vi "Dashboard Main.vi"() -> ()   [LabVIEW 2015]
uses:
  Common Code/Auton Command Cluster.ctl
  Common Code/Auton File Lists.ctl
  Vision/Camera Types.ctl
  Common Code/Goal Vision Packet.ctl
  <vilib>/Rock Robotics/WPI/Camera/WPI_CameraSettings Read MJPG.ctl
  <vilib>/Rock Robotics/WPI/Camera/WPI_CameraImageSize.ctl
  Common Code/Encoder Values Super Cluster.ctl
  Common Code/Encoder Values.ctl
  Common Code/Power and Diagnostic Data.ctl
  Common Code/Utilities/PDP Data.ctl
  Common Code/Utilities/PCM Data.ctl
  Common Code/IMU Data.ctl
  navX-MXP Library/COMMON/TypeDefs/Value TypeDefs/navX NAVX_CAL_STATUS.ctl
  navX-MXP Library/COMMON/TypeDefs/Value TypeDefs/navX NAVX_OP_STATUS.ctl
  Common Code/Intake Status Cluster.ctl
  Common Code/Intake Mode.ctl
  Common Code/Intake States.ctl
  Common Code/Climb Status Cluster.ctl
  Common Code/Climb Mode.ctl
  Common Code/Climb Presets.ctl
  Common Code/Major Loop Times.ctl
  Common Code/Shooter State Cluster.ctl
  Common Code/Shooter State.ctl
  Common Code/Shoot Modes Enum.ctl
  Common Code/Shot Type.ctl
  Common Code/Encoder Control.ctl
  Common Code/Drivetrain Status Cluster.ctl
  Common Code/Drivetrain Modes.ctl
  Common Code/Dist Drive Status.ctl
  Common Code/Drivetrain Settings.ctl
  Common Code/Shooter Presets.ctl
  Common Code/Shot Presets.ctl
  Common Code/Intake Presets.ctl
  Common Code/Drivetrain Output Range.ctl
  Common Code/Enabled Systems.ctl
  Common Code/Ultrasonic Data.ctl
  Common Code/Autonomous Presets.ctl
  Common Code/Robot Name.ctl
  Common Code/Dashboard Communication/Dashboard Control Data.ctl
  Common Code/Dashboard Drivetrain Command.ctl
  Common Code/Drivetrain Vision.ctl
  Common Code/Ball Tracking Command Cluster.ctl
  Common Code/Ball Vision Packet.ctl
  Common Code/Tracking Mode.ctl
  Common Code/IntakeEcoderControl.ctl
  Common Code/Dashboard Communication/Dashboard Display Data.ctl
  <vilib>/Rock Robotics/WPI/Dashboard/WPI_DashboardLogging Global.vi
  <vilib>/Utility/inputDevices.llb/keyboardAcquire.vi
  navX-MXP Library/navX-MXP IMU.lvlib
panel:
  in  "Robot":T1
  in  "Logging Filename":path=path ""
  in  "stop":bool
  out "DumbDashMessage":string="137 values loaded OK"
  in  "Save":bool
  in  "Load":bool
  in  "TCP":refnum<k5>
  in  "Rec Mode":enum32{"Stop", "Record", "Playback"}(radio)
  out "Image Message":string="Timeout in Camera Communications"
  in  "Dashboard Tab":T2(tab)
  out "Front Camera Display 2":T3(plugin-control)
  out "Pressure":dbl
  out "Goal Active? 2":bool
  out "Drivetrain Mode":bool
  out "Intake State":bool
  out "Right RPM":dbl(knob) scale=0.0..5000.0
  out "Left RPM":dbl(knob) scale=0.0..5000.0
  out "Mode":T4(ring)=enum."Disconnected"
  out "Shooter Mode":bool
  out "Gyro":dbl(knob) scale=0.0..360.0 scale format="%#.7g"
  out "Climb Mode":bool
  out "Intake Mode":bool
  out "Shooter State":bool
  out "Camera IP":string="0.0.0.0"
  out "Robot IP":string="0.0.0.0"
  out "Angle Ready?":bool
  out "RPM Ready?":bool
  out "Vision Ready?":bool
  out "Ball Loaded?":bool
  out "Shooter Ready?":bool
  out "Front Camera Display":T3(plugin-control)
  in  "Camera Mode":u16(ring)=3 items=["Camera Off", "USB Camera SW", "USB Camera HW", "IP Camera"]
  out "FPS":dbl
  out "Bandwidth (Mbps)":dbl
  out "NAVX_CAL_STATUS":T5 items=["IMU_CAL_STATE_MASK"=3, "IMU_CAL_INPROGRESS"=0, "IMU_CAL_ACCUMULATE"=1, "IMU_CAL_COMPLETE"=2, "MAG_CAL_COMPLETE"=4, "BARO_CAL_COMPLETE"=8]
  in  "Auton Presets":T6
  out "Auton Command Cluster":T7
  out "Auton File Lists":T8
  in  "Drivetrain Settings":T9={"Gyro Tolerance"=6.0, "Throttle Ramp (ms)"=250.0, "Angular rate compensation"=FALSE, "Throttle to Rate Scale"=0.0, "Rate compensation gain"=0.0, "Kv"=0.0, "Ka"=0.0, "Feed Forward P"=1.0, "Feed Forward D"=0.0, "Goal Vision PID gains"={"proportional gain (Kc)"=0.8, "integral time (Ti, min)"=0.05, "derivative time (Td, min)"=0.003}, "Goal Detection Window"=12.0, "Creep Rate"=0.0} {"Goal Vision PID gains"."derivative time (Td, min)" format="%.3f"; "Goal Vision PID gains"."integral time (Ti, min)" format="%.3f"; "Goal Vision PID gains"."proportional gain (Kc)" format="%.4f"}
  out "Drivetrain Status Cluster":T10 {"2nd Gear Time" scale=0.0..135.0; "1st Gear Time" scale=0.0..135.0}
  in  "Encoder Settings":T13={"Right Tick Constant"=0.002781, "Left Tick Constant"=0.002785, "Reset?"=FALSE, "Y Dist"={"PID gains"={"proportional gain (Kc)"=0.0, "integral time (Ti, min)"=0.0, "derivative time (Td, min)"=0.0}}, "Y Stop Thresh"=0.0, "Y Stop Speed"=0.0}
  in  "Goal Output Range":cluster{"output high":dbl, "output low":dbl}={"output high"=0.8, "output low"=-0.8}
  out "Encoder Values":T14
  in  "Steer PID output":cluster{"output high":dbl, "output low":dbl}
  in  "Steer PID gains":T16
  in  "Shooter Presets":T17={"Batter Shot"={"Left"=1450.0, "Right"=1450.0, "Angle"=69.0}, "Deep Middle Shot"={"Left"=0.0, "Right"=0.0, "Angle"=0.0}, "Manual Shot"={"Left"=1000.0, "Right"=1000.0, "Angle"=0.0}, "Left Ticks Per Rotation"=-409.6, "Right Ticks Per Rotation"=409.6, "Low Bar Shot"={"Left"=2100.0, "Right"=2100.0, "Angle"=42.0}, "Shooter RPM Tolerance"=100.0, "IIR Filter Power"=0.0, "Trigger Power"=0.9, "Fire from Load Delay"=250, "Max Angle"=80.0, "Min Angle"=42.0, "Angle PID gains"={"P"=1.0, "I"=0.0, "D"=0.002}, "Angle Output"={"output high"=0.5, "output low"=-0.5}, "Shooter Angle Tolerance"=3.0, "Vision Shoot x^2"=0.0, "Vision Shoot x"=0.0, "Offset Angle"=0.0, "High Goal Center Height"=97.0, "Feed Forward Max Accel"=160.57, "Feed Forward Kv"=0.000217, "Backwards Trigger"=-0.6, "Shot Finish Delay (ms)"=250.0, "Angle Max Current"=40.0, "Angle Current Trip Time"=500.0, "Intake Angle"=80.0, "Vision Shoot c"=0.0, "Reset?"=FALSE, "Servo Release Delay"=0.0, "Servo Idle Angle"=120, "Servo Hold Angle"=55, "Angle Pot x"=7.0746, "Angle Pot c"=33.439, "Ignore Angle?"=FALSE, "Manual Output?"=FALSE, "Manual Out"=0.0, "Max RPM"=4600.0, "Safty Frist Angle"=44.0, "Intake Danger Height"=35.0, "Angle Pot B"=0, "Angle Pot M"=12.0, "FF Finish RPM"=0.0, "RPM PID Right"={"P"=0.17, "I"=0.0, "D"=0.0, "FF"=0.036}, "RPM PID Left"={"P"=0.18, "I"=0.0, "D"=0.0, "FF"=0.037}, "Backwards RPM"=-300.0, "Vision RPM"=0.0} {"Angle Output"."output low" format="%.2f"; "Angle Output"."output high" format="%.2f"}
  out "Shooter State Cluster":T19 {"Trigger Output" scale=-1.0..1.0; "Angle Motor Output" scale=-1.0..1.0; "Right RPM" scale=0.0..5000.0; "Left RPM" scale=0.0..5000.0}
  in  "Intake Presets":T23={"Intake Speed"=0.8, "Outake Speed"=-0.8, "Low Height"=5.0, "Half Height"=55.0, "Full Height"=90.0, "Angle Speed"=0.0, "Angle Tolerance"=5.0, "Encoder Scale"=0.001478, "Load Height"=4.0, "Output Range"={"output high"=0.4, "output low"=-0.4}, "Rotation Power Max/Min"=0.5, "MaxCurrent"=40.0, "Intake Trip Time"=500.0, "Idle Height"=27.0, "Max Height"=90.0, "Reset Encoders?"=FALSE, "PID gains"={"proportional gain (Kc)"=1.0, "integral time (Ti, min)"=0.0, "derivative time (Td, min)"=0.003}} {"Max Height" format="%#_7g"; "Idle Height" format="%#_7g"; "Intake Trip Time" format="%#_7g"; "MaxCurrent" format="%#_7g"; "Rotation Power Max/Min" format="%#_7g"; "Load Height" format="%#_7g"; "Encoder Scale" format="%#_7g"; "Angle Tolerance" format="%#_7g"; "Angle Speed" format="%#_7g"; "Full Height" format="%#_7g"; "Half Height" format="%#_7g"; "Low Height" format="%#_7g"; "Outake Speed" format="%#_7g"; "Intake Speed" format="%#_7g"}
  out "Intake Status Cluster":T25
  in  "Climb Presets":T28={"Pull Power"=0.0, "Time to Hold"=0.0, "Extend Power"=1.0}
  out "Climb Status Cluster":T29
  in  "Pressure B":dbl
  in  "Pressure M":dbl=22.0
  out "Pressure Sensor Voltage":dbl
  out "IMU Data":T31 {"NAVX_OP_STATUS" items=["INITIALIZING", "SELFTEST_IN_PROGRESS", "ERROR", "IMU_AUTOCAL_IN_PROGRESS", "NORMAL"]; "NAVX_CAL_STATUS" items=["IMU_CAL_STATE_MASK"=3, "IMU_CAL_INPROGRESS"=0, "IMU_CAL_ACCUMULATE"=1, "IMU_CAL_COMPLETE"=2, "MAG_CAL_COMPLETE"=4, "BARO_CAL_COMPLETE"=8]}
  out "Gyro 2":dbl(knob) scale=0.0..360.0 scale format="%#.7g"
  out "Ultrasonic Data":T33
  out "Ball Cam Active?":bool
  out "Camera Display 2":T3(plugin-control)
  in  "Aspect Fudge Factor":dbl=1.0
  in  "Score Threshold 2":dbl=75.0 format="%#_13g"
  out "Goal Display":T3(plugin-control)
  out "Found Targets":T34(array[cluster]) {"Normalized Rect"."Numeric 5" format="%#_2g"; "Normalized Rect"."Numeric 3" format="%#_2g"; "Normalized Rect"."Numeric 2" format="%#_2g"; "Normalized Rect"."Numeric" format="%#_2g"}
  in  "Camera Type":T35=enum."1013"
  out "Goal Vision Packet":T36
  in  "Goal Camera Settings":T37={"fps"=30, "compression"=30, "Image Size"=enum."320x240"}
  in  "File number":i32
  in  "Use Goal File?":bool
  in  "Color Components":T39={"Hue"={110.0, 142.0}, "Sat"={138.0, 255.0}, "Val"={139.0, 198.0}} {"Val" scale=0.0..255.0; "Sat" scale=0.0..255.0; "Hue" scale=0.0..255.0 scale format="%#_3g"}
  out "Goal Active?":bool
  in  "Camera Mode 2":u16(ring) items=["Camera Off", "USB Camera SW", "USB Camera HW", "IP Camera"]
  out "FPS 2":dbl
  out "Bandwidth (Mbps) 2":dbl
  in  "Ball Camera Settings":T37={"fps"=30, "compression"=30, "Image Size"=enum."320x240"}
  out "Front Camera Display 3":T3(plugin-control)
  out "Power and Diagnostic Data":T40
  in  "Enabled Systems":T43={"Shoot"=TRUE, "Intake"=TRUE, "DT"=TRUE, "Gyro"=TRUE, "100ms"=TRUE, "US"=TRUE}
  out "Control Info":T44
  out "Status Info":T45
  out "DS TCP":T46={"Error Strings"="", "Disable Counts"={0, 0}, "Rail Faults"={0, 0, 0}, "Robot IP"="0.0.0.0", "DB Mode"=4, "Event Info"={"Name"="", "Type"=0, "Number"=0, "Replay"=0}, "Camera Addr"="0.0.0.0"}
  out "Robot Metrics":T47
  out "Loop Times":T48
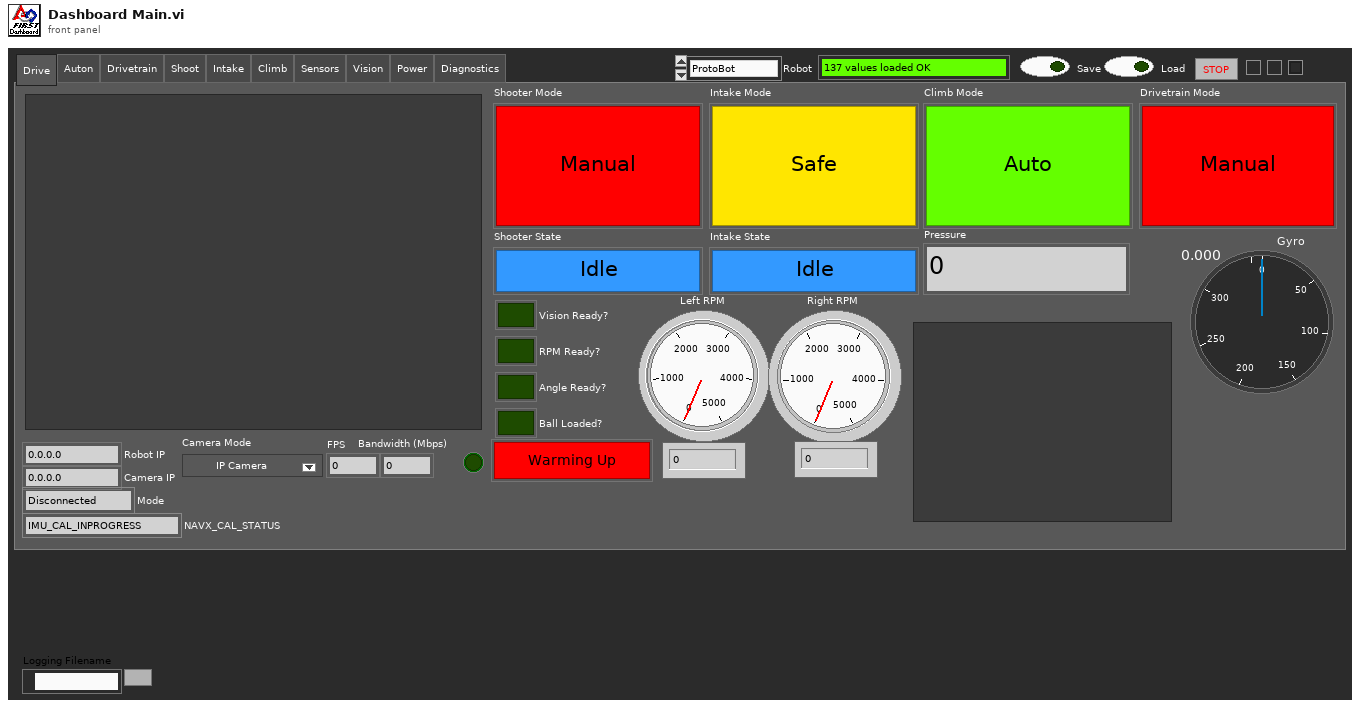
[diagram p1: front panel]
types:
  T1 = typedef "Robot Name.ctl" = enum16{"ProtoBot", "Main Robot", "Practice Robot"}
  T2 = enum32{"Drive", "Auton", "Drivetrain", "Shoot", "Intake", "Climb", "Sensors", "Vision", "Power", "Diagnostics"}
  T3 = typedef "IMAQ Image.ctl" = refnum<image>
  T4 = enum8{"Tele-Op Disabled", "Tele-Op Enabled", "Auto Disabled", "Auto Enabled", "Test Disabled", "Test Enabled", "Disconnected", "No Code", "E-Stop"}
  T5 = typedef "navX-MXP IMU.lvlib/navX NAVX_CAL_STATUS.ctl" = u8
  T6 = typedef "Autonomous Presets.ctl" = cluster{"Pitch Limit":dbl, "Roll Limit":dbl, "Ultrasonic Limit":dbl, "Start Position":dbl, "Cross Position":dbl}
  T7 = typedef "Auton Command Cluster.ctl" = cluster{"Command ID":i32, "maxTime":dbl, "Y Distance":dbl, "Heading":dbl, "Throttle":dbl, "Async":dbl, "Velocity":dbl, "Acceleration":dbl, "To":dbl, "Condition":dbl, "Shot Type":dbl, "Left RPM":dbl, "Override RPM":i32, "Override Angle":i32, "Right RPM":dbl, "Angle":dbl, "Intake Mode":i32, "Intake Cmd":i32, "Intake O":i32, "Eject O":i32, "Angle O":i32, "Arm O":i32, "Intake Speed":dbl, "Eject Speed":dbl, "Arm Angle":dbl, "Arm Speed":dbl, "Intake?":i32, "Eject?":i32, "Left":dbl, "Right":dbl, "Pivot Speed":dbl}
  T8 = typedef "Auton File Lists.ctl" = cluster{"Current Queue":string, "General Scripts":string, "Defense Scripts":string, "Movement Scripts":string}
  T9 = typedef "Drivetrain Settings.ctl" = cluster{"Gyro Tolerance":dbl, "Throttle Ramp (ms)":dbl, "Angular rate compensation":bool, "Throttle to Rate Scale":dbl, "Rate compensation gain":dbl, "Kv":dbl, "Ka":dbl, "Feed Forward P":dbl, "Feed Forward D":dbl, "Goal Vision PID gains":cluster{"proportional gain (Kc)":dbl, "integral time (Ti, min)":dbl, "derivative time (Td, min)":dbl}, "Goal Detection Window":dbl, "Creep Rate":dbl}
  T10 = typedef "Drivetrain Status Cluster.ctl" = cluster{"Modes":T11, "Y (Throttle)":dbl, "X (Steer)":dbl, "Gyro In Range?":bool, "Distance Drive Finished?":bool, "Stop Eject Lockout":bool, "Dist Drive Status":T12, "Y Target":dbl, "Heading Target":dbl, "Vision Target Aligned?":bool, "Gear":dbl, "1st Gear Time":dbl, "2nd Gear Time":dbl, "1st Gear Shifts":dbl, "2nd Gear Shifts":dbl}
  T11 = typedef "Drivetrain Modes.ctl" = enum16{"Tank", "Climb", "Manual", "Goal Vision Targeting", "PID Distance Drive", "Hybrid", "Gyro Steer"}
  T12 = typedef "Dist Drive Status.ctl" = cluster{"Y In Range":bool, "X In Range":bool, "Gyro In Range":bool, "Y Dist":dbl, "X Dist":dbl, "Gyro":dbl}
  T13 = typedef "Encoder Control.ctl" = cluster{"Right Tick Constant":dbl, "Left Tick Constant":dbl, "Reset?":bool, "Y Dist":cluster{"PID gains":cluster{"proportional gain (Kc)":dbl, "integral time (Ti, min)":dbl, "derivative time (Td, min)":dbl}}, "Y Stop Thresh":dbl, "Y Stop Speed":dbl}
  T14 = typedef "Encoder Values Super Cluster.ctl" = cluster{"Left Encoder":T15, "Right Encoder":T15}
  T15 = typedef "Encoder Values.ctl" = cluster{"Distance":dbl, "Speed":dbl, "Ticks":dbl}
  T16 = cluster{"proportional gain (Kc)":dbl, "integral time (Ti, min)":dbl, "derivative time (Td, min)":dbl}
  T17 = typedef "Shooter Presets.ctl" = cluster{"Batter Shot":T18, "Deep Middle Shot":T18, "Manual Shot":T18, "Left Ticks Per Rotation":dbl, "Right Ticks Per Rotation":dbl, "Low Bar Shot":T18, "Shooter RPM Tolerance":dbl, "IIR Filter Power":dbl, "Trigger Power":dbl, "Fire from Load Delay":i32, "Max Angle":dbl, "Min Angle":dbl, "Angle PID gains":cluster{"P":dbl, "I":dbl, "D":dbl}, "Angle Output":cluster{"output high":dbl, "output low":dbl}, "Shooter Angle Tolerance":dbl, "Vision Shoot x^2":dbl, "Vision Shoot x":dbl, "Offset Angle":dbl, "High Goal Center Height":dbl, "Feed Forward Max Accel":dbl, "Feed Forward Kv":dbl, "Backwards Trigger":dbl, "Shot Finish Delay (ms)":dbl, "Angle Max Current":dbl, "Angle Current Trip Time":dbl, "Intake Angle":dbl, "Vision Shoot c":dbl, "Reset?":bool, "Servo Release Delay":dbl, "Servo Idle Angle":i32, "Servo Hold Angle":i32, "Angle Pot x":dbl, "Angle Pot c":dbl, "Ignore Angle?":bool, "Manual Output?":bool, "Manual Out":dbl, "Max RPM":dbl, "Safty Frist Angle":dbl, "Intake Danger Height":dbl, "Angle Pot B":i32, "Angle Pot M":dbl, "FF Finish RPM":dbl, "RPM PID Right":cluster{"P":dbl, "I":dbl, "D":dbl, "FF":dbl}, "RPM PID Left":cluster{"P":dbl, "I":dbl, "D":dbl, "FF":dbl}, "Backwards RPM":dbl, "Vision RPM":dbl}
  T18 = typedef "Shot Presets.ctl" = cluster{"Left":dbl, "Right":dbl, "Angle":dbl}
  T19 = typedef "Shooter State Cluster.ctl" = cluster{"State":T20, "Left RPM":dbl, "Right RPM":dbl, "Shooter Ready?":bool, "Ball Loaded?":bool, "Current Angle":dbl, "Angle Motor Output":dbl, "Trigger Output":dbl, "Angle Ready?":bool, "RPM Ready?":bool, "Vision Ready?":bool, "Ball Loaded?":bool, "Mode":T21, "Shot Type":T22, "Pot Height":dbl, "Current Tripped Forward?":bool, "Current Tripped Backward?":bool, "Right Servo":i32, "Left Servo":i32, "IR Override":bool, "Intake Danger?":bool}
  T20 = typedef "Shooter State.ctl" = enum16{"Idle", "Warmup", "Shooter Ready", "Shoot"}
  T21 = typedef "Shoot Modes Enum.ctl" = enum16{"Manual", "Safe", "Auto"}
  T22 = typedef "Shot Type.ctl" = enum16{"Batter Shot", "Corner Shot", "Curve Shot", "Vision Shot", "Deep Middle Shot"}
  T23 = typedef "Intake Presets.ctl" = cluster{"Intake Speed":dbl, "Outake Speed":dbl, "Low Height":dbl, "Half Height":dbl, "Full Height":dbl, "Angle Speed":dbl, "Angle Tolerance":dbl, "Encoder Scale":dbl, "Load Height":dbl, "Output Range":T24, "Rotation Power Max/Min":dbl, "MaxCurrent":dbl, "Intake Trip Time":dbl, "Idle Height":dbl, "Max Height":dbl, "Reset Encoders?":bool, "PID gains":cluster{"proportional gain (Kc)":dbl, "integral time (Ti, min)":dbl, "derivative time (Td, min)":dbl}}
  T24 = typedef "Drivetrain Output Range.ctl" = cluster{"output high":dbl, "output low":dbl}
  T25 = typedef "Intake Status Cluster.ctl" = cluster{"Roller Power":dbl, "Angle Power":dbl, "Intake Mode":T26, "Intake States":T27, "Rollers Active?":bool, "Current Height":dbl, "Target Height":dbl, "Encoder Raw Position":dbl, "Forward Tripped?":bool, "Backward Tripped?":bool, "Override IR?":bool}
  T26 = typedef "Intake Mode.ctl" = enum16{"Safe", "Auto", "Manual"}
  T27 = typedef "Intake States.ctl" = enum16{"Idle", "Set roller speed", "Move to angle"}
  T28 = typedef "Climb Presets.ctl" = cluster{"Pull Power":dbl, "Time to Hold":dbl, "Extend Power":dbl}
  T29 = typedef "Climb Status Cluster.ctl" = cluster{"Pull Power":dbl, "Unpin Power":dbl, "PTO Engaged?":bool, "Climb Mode":T30}
  T30 = typedef "Climb Mode.ctl" = enum16{"Auto", "Semi-Auto", "Manual"}
  T31 = typedef "IMU Data.ctl" = cluster{"Pitch":sgl, "Roll":sgl, "Yaw":sgl, "Data Valid?":bool, "Temp":sgl, "MOVING":bool, "YAW_STABLE":bool, "Accel X":sgl, "Accel Y":sgl, "Accel Z":sgl, "Accel Magnitude":sgl, "Pitch Rate":sgl, "Roll Rate":sgl, "Yaw Rate":sgl, "NavX Opened?":bool, "NAVX_CAL_STATUS":T5, "NAVX_OP_STATUS":T32}
  T32 = typedef "navX-MXP IMU.lvlib/navX NAVX_OP_STATUS.ctl" = u8
  T33 = typedef "Ultrasonic Data.ctl" = cluster{"Left Ultrasonic":dbl, "Right Ultrasonic":dbl}
  T34 = cluster{"Distance (ft)":dbl, "Center":cluster{dbl, dbl}, "Normalized Rect":cluster{"Numeric":dbl, "Numeric 2":dbl, "Numeric 3":dbl, "Numeric 5":dbl}}[]
  T35 = typedef "Camera Types.ctl" = enum16{"206", "1011", "1013", "MS HD3000 square", "MS HD3000 640x480"}
  T36 = typedef "Goal Vision Packet.ctl" = cluster{"Distance":dbl, "Center X":dbl, "Center Y":dbl, "Found Target?":bool, "Robot Center":dbl, "Angle":dbl}
  T37 = typedef "WPI_CameraSettings Read MJPG.ctl" = cluster{"fps":i32, "compression":i32, "Image Size":T38}
  T38 = typedef "WPI_CameraImageSize.ctl" = enum16{"640x480", "320x240", "160x120", "Custom"}
  T39 = cluster{"Hue":cluster{dbl, dbl}, "Sat":cluster{dbl, dbl}, "Val":cluster{dbl, dbl}}
  T40 = typedef "Power and Diagnostic Data.ctl" = cluster{"PDP Data":T41, "PCM Data":T42, "roboRIO input voltage (V)":dbl, "roboRIO input current (A)":dbl, "3.3V Rail Short":bool, "5 V Rail Short":bool, "6 V Rail Short":bool, "roboRIO Brownout":bool, "Outputs Enabled?":bool}
  T41 = typedef "PDP Data.ctl" = cluster{"Battery Voltage":sgl, "Temperature (degrees C)":sgl, "Internal Battery R (Ohms)":sgl, "Energy (J)":sgl, "Power (W)":sgl, "Total Current (A)":sgl, "Battery Voltage Fault":bool, "Temperature Fault":bool, "Hardware Fault":bool, "Currents":cluster{"[0]":sgl, "[1]":sgl, "[2]":sgl, "[3]":sgl, "[4]":sgl, "[5]":sgl, "[6]":sgl, "[7]":sgl, "[8]":sgl, "[9]":sgl, "[10]":sgl, "[11]":sgl, "[12]":sgl, "[13]":sgl, "[14]":sgl, "[15]":sgl}, "Current Faults":cluster{"[0]":bool, "[1]":bool, "[2]":bool, "[3]":bool, "[4]":bool, "[5]":bool, "[6]":bool, "[7]":bool, "[8]":bool, "[9]":bool, "[10]":bool, "[11]":bool, "[12]":bool, "[13]":bool, "[14]":bool, "[15]":bool}}
  T42 = typedef "PCM Data.ctl" = cluster{"Compressor Fault":bool, "Solenoid Fault":bool, "Compressor Enabled":bool, "Hardware Fault":bool, "Compressor Current":dbl}
  T43 = typedef "Enabled Systems.ctl" = cluster{"Shoot":bool, "Intake":bool, "DT":bool, "Gyro":bool, "100ms":bool, "US":bool}
  T44 = cluster{"Control Bits":cluster{"TestMode":bool, "Autonomous":bool, "Enabled":bool, "FMS Present":bool, bool, bool, bool, "E-Stop":bool}, "Team Station ":u8, "Countdown":sgl, "Joystick Values":cluster{"Axes":dbl[], "Buttons":bool[], "POVs":i16[]}[]}
  T45 = cluster{"Status bits":cluster{"Test Mode":bool, "Autonomous":bool, "Enabled":bool, "Code Start":bool, "Brownout":bool, "Reserved 2":bool, "Reserved 3":bool, "E-Stop":bool}, "Code Trace":cluster{"Disabled":bool, "TeleOp":bool, "Auto":bool, "Test":bool}, "Controller Type":enum16{"unknown", "cRIO", "roboRio"}, "Code?":enum16{"unknown", "noCode", "code"}, "Battery V":dbl}
  T46 = cluster{"Error Strings":string, "Disable Counts":cluster{u16, u16}, "Rail Faults":cluster{u16, u16, u16}, "Robot IP":string, "DB Mode":u8, "Event Info":cluster{"Name":string, "Type":u8, "Number":u16, "Replay":u8}, "Camera Addr":string}
  T47 = cluster{"Storage":cluster{"Disk Free":u64, "RAM Block":u32, "RAM free":u32}, "CPU Utilization":cluster{"CPU % ISR":sgl, "CPU % Time Crit":sgl, "CPU % Timed Str":sgl, "CPU % High":sgl, "CPU % Above":sgl, "CPU % Normal":sgl, "CPU % Low":sgl}, "CAN":cluster{"% Bus Utilization":sgl, "Bus Off Cnt":u32, "TX_FIFO Full Cnt":u32, "Receive Error Cnt":u8, "Transmit Error Cnt":u8}, "HID":cluster{"HID Outputs":u32, "Rumble Low":u16, "Rumble High":u16}[]}
  T48 = typedef "Major Loop Times.ctl" = cluster{"DT Loop Timer":u32, "Shooter Loop Timer":u32, "Intake Loop Timer":u32, "US Loop Timer":u32, "Auton File Loop Timer":u32}
  T49 = typedef "Image Type" = u32
  T50 = typedef "NI_LVConfig.lvlib/Config Data RefNum.ctl" = refnum<k1>
  T51 = cluster{cluster{dbl, dbl}, cluster{dbl, dbl}, cluster{dbl, dbl}}
  T52 = cluster{"Bounding box":cluster{"left":dbl, "top":dbl, "right":dbl, "bottom":dbl}, "Aspect Ratio":dbl, "Area to CH":dbl, "X Mask":dbl, "Y Mask":dbl, "Moment":dbl}[]
  T53 = cluster{"Distance (ft)":dbl, "Center":cluster{dbl, dbl}, "Normalized Rect":cluster{"Numeric":dbl, "Numeric 2":dbl, "Numeric 3":dbl, "Numeric 5":dbl}}
  T54 = typedef "Dashboard Display Data.ctl" = cluster{"Auton Command Cluster":T7, "Auton File Lists":T8, "Drivetrain Status Cluster":T10, "Encoder Values":T14, "IMU Data":T31, "Power and Diagnostic Data":T40, "Gyro":dbl, "Shooter State Cluster":T19, "Intake Status Cluster":T25, "Ultrasonic Data":T33, "Climb Status Cluster":T29, "Loop Times":T48, "Pressure":dbl, "Pressure Voltage":dbl}
  T55 = typedef "Dashboard Control Data.ctl" = cluster{"Shooter Presets":T17, "Encoder Control":T13, "Steer PID output":cluster{"output high":dbl, "output low":dbl}, " Steer PID gains":cluster{"proportional gain (Kc)":dbl, "integral time (Ti, min)":dbl, "derivative time (Td, min)":dbl}, "Drivetrain Settings":T9, "Vision Packet":T36, "Dashboard Drivetrain Command":T56, "Info/Command Cluster":T58, "Ball Vision Packet":T59, "Intake Presets":T23, "Intake Encoder Control":T61, "Climb Presets":T28, "Goal Output Range":cluster{"output high":dbl, "output low":dbl}, "Enabled Systems":T43, "Auton Presets":T6, "Pressure M":dbl, "Pressure B":dbl}
  T56 = typedef "Dashboard Drivetrain Command.ctl" = cluster{"Drivetrain Vision":T57}
  T57 = typedef "Drivetrain Vision.ctl" = cluster{"Goal Window":dbl, "Ball Window":dbl}
  T58 = typedef "Ball Tracking Command Cluster.ctl" = cluster{"Distance to Ball":dbl, "Desired Angle":dbl, "Command":enum16{"Turn to Ball", "Turn to Angle", "Get Distance"}, "Pixels from Center":dbl}
  T59 = typedef "Ball Vision Packet.ctl" = cluster{"Ball Detected?":bool, "Distance to Ball":dbl, "Desired Angle":dbl, "Pixels from Center":dbl, "Tracking mode":T60}
  T60 = typedef "Tracking Mode.ctl" = enum16{"Turn to Ball", "Turn to Angle"}
  T61 = typedef "IntakeEcoderControl.ctl" = cluster{"Arm Tick Constant":dbl, "Reset?":bool, "Y Dist":cluster{"PID gains":cluster{"proportional gain (Kc)":dbl, "integral time (Ti, min)":dbl, "derivative time (Td, min)":dbl}}, "Y Stop Thresh":dbl, "Y Stop Speed":dbl}
  T62 = cluster{"Image Size":bool, "Image Type":bool, "Pixel Value":bool, "ROI Information":bool, "Zoom Factor":bool}
  T63 = enum16{"0", "1", "2", "3", "4", "5", "6", "7", "8", "9", "A", "B", "C", "D", "E", "F", "G", "H", "I", "J", "K", "L", "M", "N", "O", "P", "Q", "R", "S", "T", "U", "V", "W", "X", "Y", "Z", "F1", "F2", "F3", "F4", "F5", "F6", "F7", "F8", "F9", "F10", "F11", "F12", "F13", "F14", "F15", "ADD", "BACK", "BACKSLASH", "CAPITAL", "COMMA", "DECIMAL", "DELETE", "DIVIDE", "DOWN", "END", "EQUALS", "ESCAPE", "GRAVE (`)", "HOME", "INSERT", "LBRACKET", "LCONTROL", "LEFT", "L ALT", "LSHIFT", "LWIN", "MINUS", "MULTIPLY", "NEXT", "NUMLOCK", "NUMPAD_0", "NUMPAD_1", "NUMPAD_2", "NUMPAD_3", "NUMPAD_4", "NUMPAD_5", "NUMPAD_6", "NUMPAD_7", "NUMPAD_8", "NUMPAD_9", "PAUSE", "PERIOD", "PRIOR (PG UP)", "RBRACKET", "RCONTROL", "RETURN", "RIGHT", "R ALT", "RSHIFT", "RWIN", "SCROLL", "SEMICOLON", "SLASH", "SPACE", "SUBTRACT", "TAB", "UP", "ENTER (num pad)", "' (quote)"}[]
  T64 = typedef "DumbDash Control.ctl" = cluster{"Name":string, "Ref":refnum<vi>, "Type":T65}
  T65 = typedef "DumbDash Control Type.ctl" = enum16{"Invalid", "Number", "Boolean", "String"}
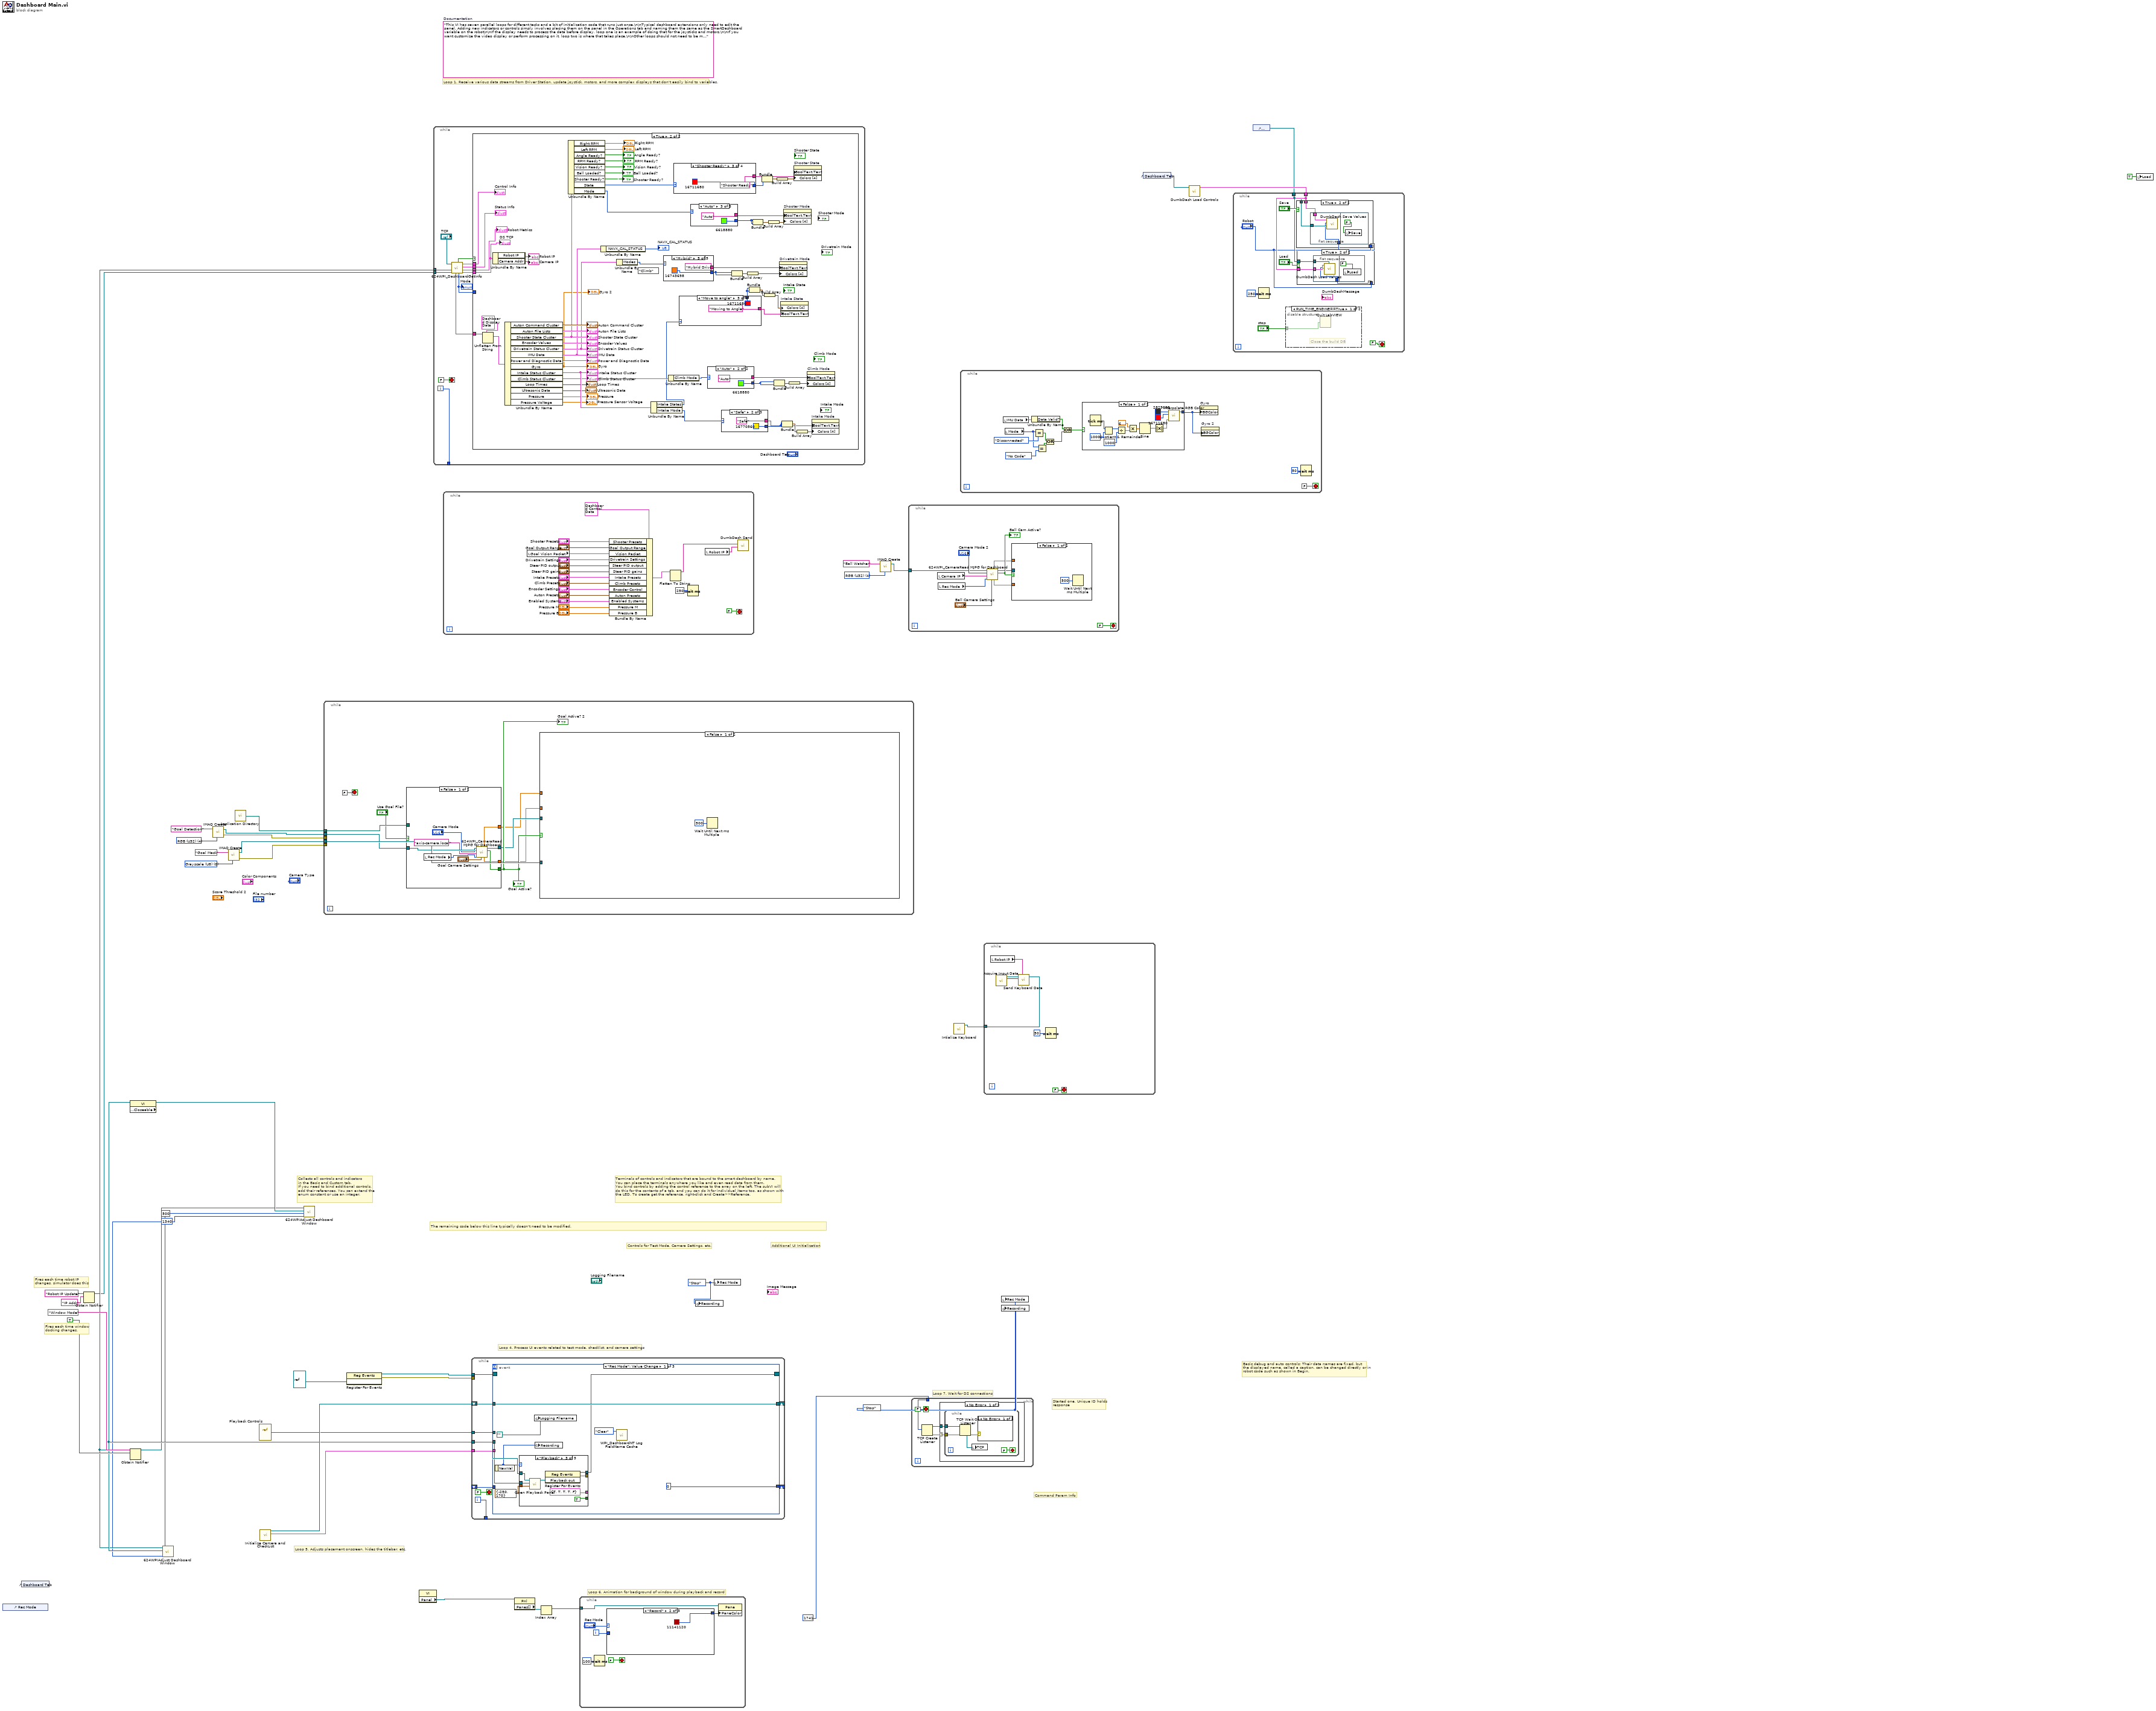
[diagram p0: block diagram]
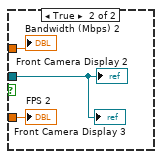
[diagram p2: hidden frame]
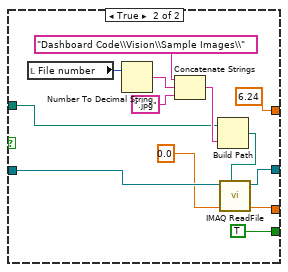
[diagram p3: hidden frame]
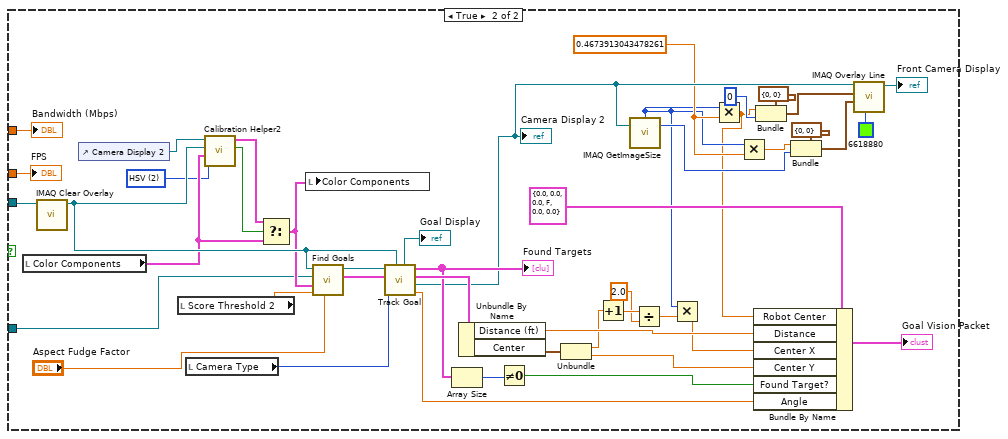
[diagram p4: hidden frame]
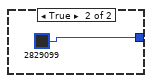
[diagram p5: hidden frame]
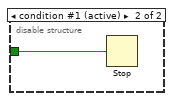
[diagram p6: hidden frame]
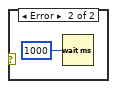
[diagram p9: hidden frame]
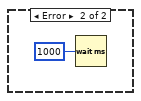
[diagram p10: hidden frame]
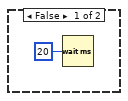
[diagram p11: hidden frame]
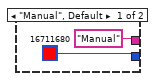
[diagram p12: hidden frame]
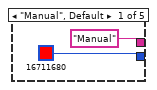
[diagram p13: hidden frame]
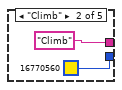
[diagram p14: hidden frame]
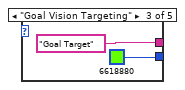
[diagram p15: hidden frame]
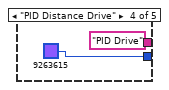
[diagram p16: hidden frame]
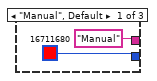
[diagram p17: hidden frame]
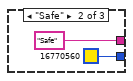
[diagram p18: hidden frame]
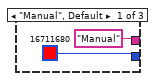
[diagram p19: hidden frame]
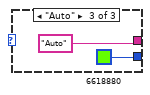
[diagram p20: hidden frame]
diagram:
  w4 = T49 4 items=["Grayscale (U8)", "Grayscale (I16)", "Grayscale (SGL)", "Complex (CSG)", "RGB (U32)", "HSL (U32)", "RGB (U64)", "Grayscale (U16)"] ("Image Type")
  w6 = T49 0 items=["Grayscale (U8)", "Grayscale (I16)", "Grayscale (SGL)", "Complex (CSG)", "RGB (U32)", "HSL (U32)", "RGB (U64)", "Grayscale (U16)"] ("Image Type")
  w11 = T49 4 items=["Grayscale (U8)", "Grayscale (I16)", "Grayscale (SGL)", "Complex (CSG)", "RGB (U32)", "HSL (U32)", "RGB (U64)", "Grayscale (U16)"] ("Image Type")
  w15 = enum16{"Stop", "Record", "Playback"}."Stop"
  w20 = 1340
  w21 = 500
  w25 = enum32{"Stop", "Record", "Playback"}."Stop" ("Rec Mode")
  (unwired) "This VI has seven parallel loops for different tasks and a bit of initialization code that runs just once.\n\nTypical dashboard extensions only need to edit the panel. Adding new indicators or controls simply involves placing them on the panel in the Operations tab and naming them the same as the SmartDashboard variable on the robot\n\nIf the display needs to process the data before display, loop one is an example of doing that for the joysticks and motors.\n\nIf you want customize the video display or perform processing on it, loop two is where that takes place.\n\nOther loops should not need to be modified. They are pretty standard, and document the task they perform."  # Documentation
  # "Command Param Info"
  # "Started one, Unique ID holds\nresponse"
  # "Loop 7. Wait for DS connections"
  # "Basic debug and auto controls: Their data names are fixed, but\nthe displayed name, called a caption, can be changed directly or in\nrobot code such as shown in Begin."
  # "Controls for Test Mode, Camera Settings, etc."
  # "Additional UI Initialization"
  # "Loop 6. Animation for background of window during playback and record"
  # "Fires each time robot IP\nchanges, simulator does this"
  # "Fires each time window\ndocking changes."
  # "Collects all controls and indicators\nin the Basic and Custom tab.\nIf you need to bind additional controls,\nadd their references. You can extend the\nenum constant or use an integer."
  # "The remaining code below this line typically doesn't need to be modified."
  # "Loop 4. Process UI events related to test mode, checklist, and camera settings"
  # "Terminals of controls and indicators that are bound to the smart dashboard by name.\nYou can place the terminals anywhere you like and even read data from them.\nYou bind controls by adding the control reference to the array on the left. The subVI will\ndo this for the contents of a tab, and you can do it for individual items too, as shown with\nthe LED. To create get the reference, right-click and Create>>Reference."
  # "Loop 5. Adjusts placement onscreen, hides the titlebar, etc."
  # "Loop 1. Receive various data streams from Driver Station, update joystick, motors, and more complex displays that don't easily bind to variables."
  n1 = control-ref of="Rec Mode"() -> ()  [unwired: 1 out]
  n2 = control-ref of="Dashboard Tab"() -> ()  [unwired: 1 out]
  n3 = Obtain Notifier(name (unnamed)="Robot IP Update", notification data type="IP Addr" ("name (unnamed)")) -> (notifier out=w19:refnum<notifier>)  [unwired: 2 in, 2 out]
  n4 = property class="VI" props=["Front Panel.Closeable"]() -> (reference out=w24:refnum<vi>)  [unwired: 2 in, 2 out]
  n5 = Obtain Notifier(name (unnamed)="Window Mode", notification data type=TRUE) -> (notifier out=w23:refnum<notifier>)  [unwired: 2 in, 2 out]
  n6 = call "624WPIAdjust Dashboard Window.vi"("Width"=w20, "Height"=w21, "VI"=w24, "Notifier in"=w23) -> ()  [unwired: 8 in]
  n7 = call "IMAQ Create"("Image Name"="Goal Detection", "Image Type"=w11) -> ("New Image"=w13:T3, "error out"=w12:errorcluster)  [unwired: 3 in]
  n8 = call "IMAQ Create"("Image Name"="Goal Mask", "Image Type"=w6) -> ("New Image"=w9:T3, "error out"=w8:errorcluster)  [unwired: 3 in]
  n9 = call <vilib>:"Application Directory.vi"() -> ("Application Directory"=w5:path)
  n10 = vi-ref "Playback Controls.vi"() -> (w29:refnum<vi>)
  n11 = call "Initialize Camera and CheckList.vi"() -> ("Array"=w34:cluster{string[]}[], "File Refnum"=w33:T50)  [unwired: 9 in, 1 out]
  n12 = call "624WPIAdjust Dashboard Window.vi"("Width"=w20, "Height"=w21, "VI"=w24, "Notifier in"=w23) -> ()  [unwired: 8 in]
  n13 = while {
    tunnel: w12 -> [_]
    tunnel: w9 -> [w47]
    tunnel: w8 -> [_]
    tunnel: w13 -> [w45]
    tunnel: w5 -> [w43]
    stop <- FALSE stop-if-true
    n14 = case shown="False" "Use Goal File?" {
      tunnel: [w51 TRUE] -> w46
      tunnel: w45 -> [w56 w67]
      tunnel: [w50 w66] -> w44
      tunnel: w43 -> [_ w61]
      tunnel: [w48 6.24 ("Bandwidth (Mbps)")] -> w41
      tunnel: [w49 0.0 ("FPS")] -> w40
      frame False {
        n15 = local read "Rec Mode"() -> (w53:enum32{"Stop", "Record", "Playback"})
        n16 = call "624WPI_CameraRead MJPG for Dashboard.vi"("Camera Settings"="Goal Camera Settings", "Rec Mode"=w53, "Camera IP"="axis-camera.local", "Camera Mode"="Camera Mode", "Refnum in"=w56) -> ("Active"=w51:bool, "Refnum out"=w50:T3, "FPS"=w49:dbl, "Bandwidth (Mbps)"=w48:dbl)  [unwired: 3 in]
      }
      frame True {
        n17 = local read "File number"() -> (w59:i32)
        n18 = Number To Decimal String(number=w59) -> (decimal integer string=w64:string)  [unwired: 1 in]
        n19 = Concatenate Strings("Dashboard Code\\Vision\\Sample Images\\", w64, ".jpg" ("string")) -> (w62:string)
        n20 = Build Path(base path=w61, name or relative path=w62) -> (appended path=w60:path)
        n21 = call "IMAQ ReadFile"("File Path"=w60, "Image"=w67) -> ("Image Out"=w66:T3)  [unwired: 5 in, 4 out]
      }
    }
    "Goal Active?" <- w46
    "Goal Active? 2" <- w46
    n22 = case shown="False" w46 {
      tunnel: w44 -> [_ w113]
      tunnel: w47 -> [_ w90]
      tunnel: w41 -> [_ w100]
      tunnel: w40 -> [_ w99]
      frame False {
        n23 = Wait Until Next ms Multiple(millisecond multiple=u32 500) -> ()  [unwired: 1 out]
      }
      frame True {
        w80 = 0.4673913043478261
        w93 = u16 2 items=["RGB", "HSL", "HSV", "HSI", "CIE L*a*b*", "CIE XYZ"] ("Color Mode")
        n24 = local read "Color Components"() -> (w94:T39)
        n25 = call "IMAQ Clear Overlay"("Image"=w113) -> ("Image Out"=w98:T3)  [unwired: 9 in, 1 out]
        n26 = control-ref of="Camera Display 2"() -> (w97:refnum<vi>)
        n27 = local read "Score Threshold 2"() -> (w114:dbl)
        n28 = local read "Camera Type"() -> (w110:T35)
        n29 = call "Calibration Helper2.vi"("Color Mode"=w93, "Color Components"=w94, "Image"=w98, "Image Ctl Refnum"=w97) -> ("Changed"=w96:bool, "output color"=w95:T51)  [unwired: 6 in]
        n30 = Select(t=w95, s=w96, f=w94) -> (s? t:f=w92:T39)
        n31 = local write "Color Components"(w92) -> ()
        n32 = call "Find Goals.vi"("Aspect Fudge Factor"="Aspect Fudge Factor", "Score Threshold"=w114, "Color"=w92, "Image Dst"=w90, "Image Src"=w98) -> ("Targets"=w112:T52, "Masked Image"=w111:T3)  [unwired: 5 in]
        n33 = call "Track Goal.vi"("Original Image"=w98, "Camera Type"=w110, "Targets"=w112, "Goal Display"=w111) -> ("Angle Difference"=w72:dbl, "Target Line Masking Out"=w81:T3, "Best Target Available"=w109:T53, "Found Targets"=w102:T34, "Goal Display"=→"Goal Display":T3)  [unwired: 3 in]
        "Found Targets" <- w102
        "Camera Display 2" <- w81
        n34 = Array Size(array=w102) -> (size(s)=w103:i32)
        n35 = Unbundle By Name(w109) -> ("Distance (ft)"=w107:dbl, "Center"=w106:cluster{dbl, dbl})
        n36 = Not Equal To 0?(x=w103) -> (x != 0?=w101:bool)
        n37 = Unbundle(w106) -> (w79:dbl, w105:dbl)
        n38 = Increment(x=w79) -> (x+1=w78:dbl)
        n39 = call "IMAQ GetImageSize"("Image"=w81) -> ("Y Resolution"=w83:i32, "X Resolution"=w74:i32)  [unwired: 3 in, 1 out]
        n40 = Divide(x=w78, y=2.0) -> (x/y=w76:dbl)
        n41 = Multiply(x=w74, y=w76) -> (x*y=w75:dbl)
        n42 = Multiply(x=w74, y=w80) -> (x*y=w73:dbl)
        n43 = Multiply(x=w74, y=w80) -> (x*y=w86:dbl)
        n44 = Bundle By Name(cluster=T36 {"Distance"=0.0, "Center X"=0.0, "Center Y"=0.0, "Found Target?"=FALSE, "Robot Center"=0.0, "Angle"=0.0}, "Robot Center"=w73, "Distance"=w107, "Center X"=w75, "Center Y"=w105, "Found Target?"=w101, "Angle"=w72) -> (→"Goal Vision Packet":T36)
        n45 = Bundle(cluster=cluster{"X":i32, "Y":i32} {"X"=0, "Y"=0} ("Start Point"), "X"=w73, "Y"=0) -> (w85:cluster{"X":i32, "Y":i32})
        n46 = Bundle(cluster=cluster{"X":i32, "Y":i32} {"X"=0, "Y"=0} ("Start Point"), "X"=w86, "Y"=w83) -> (w84:cluster{"X":i32, "Y":i32})
        n47 = call "IMAQ Overlay Line"("Color"=u32 6618880, "End Point"=w84, "Start Point"=w85, "Image"=w81) -> ("Image Out"=→"Front Camera Display":T3)  [unwired: 6 in, 1 out]
        "Bandwidth (Mbps)" <- w100
        "FPS" <- w99
      }
    }
  }
  n48 = register-events(refnum<vi> refnum) -> (reference out=w28:refnum<event-registration>, error out=w27:errorcluster)  [unwired: 2 in]
  n49 = property class="VI"() -> ("Panel"=w31:refnum<vi>)  [unwired: 2 in, 2 out]
  n50 = while {
    tunnel: [w125] -> _
    tunnel: w19 -> [w124]
    tunnel: w23 -> [w122]
    i -> [w125]
    stop <- FALSE stop-if-true
    n51 = call "624WPI_DashboardGetInfo.vi"("Binding Refnum"=w124, "Window Mode Notifier"=w122, "TCP Cnx"="TCP") -> ("Power and Errors"=w121:T46, "Robot Metrics"=w120:T47, "Status Info"=w119:T45, "Control Info"=w118:T44, "Robot Mode"=w117:T4, "Process?"=w116:bool, "Custom Dashboard Data"=w115:string)  [unwired: 2 in]
    "Mode" <- w117
    n52 = case shown="True" w116 {
      tunnel: w119 -> [_ w187]
      tunnel: w120 -> [_ w186]
      tunnel: w118 -> [_ w188]
      tunnel: w121 -> [_ w185]
      tunnel: w117 -> [_ _]
      tunnel: w115 -> [_ w182]
      frame False {
        n53 = Wait (ms)(milliseconds to wait=u32 20) -> ()  [unwired: 1 out]
      }
      frame True {
        (unwired) Drivetrain_Modes."Climb" ("Modes")
        n54 = Unflatten From String(type=T54 {"Auton Command Cluster"={"Command ID"=0, "maxTime"=0.0, "Y Distance"=0.0, "Heading"=0.0, "Throttle"=0.0, "Async"=0.0, "Velocity"=0.0, "Acceleration"=0.0, "To"=0.0, "Condition"=0.0, "Shot Type"=0.0, "Left RPM"=0.0, "Override RPM"=0, "Override Angle"=0, "Right RPM"=0.0, "Angle"=0.0, "Intake Mode"=0, "Intake Cmd"=0, "Intake O"=0, "Eject O"=0, "Angle O"=0, "Arm O"=0, "Intake Speed"=0.0, "Eject Speed"=0.0, "Arm Angle"=0.0, "Arm Speed"=0.0, "Intake?"=0, "Eject?"=0, "Left"=0.0, "Right"=0.0, "Pivot Speed"=0.0}, "Auton File Lists"={"Current Queue"="", "General Scripts"="", "Defense Scripts"="", "Movement Scripts"=""}, "Drivetrain Status Cluster"={"Modes"=enum."Manual", "Y (Throttle)"=0.0, "X (Steer)"=0.0, "Gyro In Range?"=FALSE, "Distance Drive Finished?"=FALSE, "Stop Eject Lockout"=FALSE, "Dist Drive Status"={"Y In Range"=FALSE, "X In Range"=FALSE, "Gyro In Range"=FALSE, "Y Dist"=0.0, "X Dist"=0.0, "Gyro"=0.0}, "Y Target"=0.0, "Heading Target"=0.0, "Vision Target Aligned?"=FALSE, "Gear"=0.0, "1st Gear Time"=0.0, "2nd Gear Time"=0.0, "1st Gear Shifts"=0.0, "2nd Gear Shifts"=0.0}, "Encoder Values"={"Left Encoder"={"Distance"=0.0, "Speed"=0.0, "Ticks"=0.0}, "Right Encoder"={"Distance"=0.0, "Speed"=0.0, "Ticks"=0.0}}, "IMU Data"={"Pitch"=0.0, "Roll"=0.0, "Yaw"=0.0, "Data Valid?"=FALSE, "Temp"=0.0, "MOVING"=FALSE, "YAW_STABLE"=FALSE, "Accel X"=0.0, "Accel Y"=0.0, "Accel Z"=0.0, "Accel Magnitude"=0.0, "Pitch Rate"=0.0, "Roll Rate"=0.0, "Yaw Rate"=0.0, "NavX Opened?"=FALSE, "NAVX_CAL_STATUS"=0, "NAVX_OP_STATUS"=0}, "Power and Diagnostic Data"={"PDP Data"={"Battery Voltage"=0.0, "Temperature (degrees C)"=0.0, "Internal Battery R (Ohms)"=0.0, "Energy (J)"=0.0, "Power (W)"=0.0, "Total Current (A)"=0.0, "Battery Voltage Fault"=FALSE, "Temperature Fault"=FALSE, "Hardware Fault"=FALSE, "Currents"={"[0]"=0.0, "[1]"=0.0, "[2]"=0.0, "[3]"=0.0, "[4]"=0.0, "[5]"=0.0, "[6]"=0.0, "[7]"=0.0, "[8]"=0.0, "[9]"=0.0, "[10]"=0.0, "[11]"=0.0, "[12]"=0.0, "[13]"=0.0, "[14]"=0.0, "[15]"=0.0}, "Current Faults"={"[0]"=FALSE, "[1]"=FALSE, "[2]"=FALSE, "[3]"=FALSE, "[4]"=FALSE, "[5]"=FALSE, "[6]"=FALSE, "[7]"=FALSE, "[8]"=FALSE, "[9]"=FALSE, "[10]"=FALSE, "[11]"=FALSE, "[12]"=FALSE, "[13]"=FALSE, "[14]"=FALSE, "[15]"=FALSE}}, "PCM Data"={"Compressor Fault"=FALSE, "Solenoid Fault"=FALSE, "Compressor Enabled"=FALSE, "Hardware Fault"=FALSE, "Compressor Current"=0.0}, "roboRIO input voltage (V)"=0.0, "roboRIO input current (A)"=0.0, "3.3V Rail Short"=FALSE, "5 V Rail Short"=FALSE, "6 V Rail Short"=FALSE, "roboRIO Brownout"=FALSE, "Outputs Enabled?"=FALSE}, "Gyro"=0.0, "Shooter State Cluster"={"State"=enum."Idle", "Left RPM"=0.0, "Right RPM"=0.0, "Shooter Ready?"=FALSE, "Ball Loaded?"=FALSE, "Current Angle"=0.0, "Angle Motor Output"=0.0, "Trigger Output"=0.0, "Angle Ready?"=FALSE, "RPM Ready?"=FALSE, "Vision Ready?"=FALSE, "Ball Loaded?"=FALSE, "Mode"=enum."Manual", "Shot Type"=enum."Batter Shot", "Pot Height"=0.0, "Current Tripped Forward?"=FALSE, "Current Tripped Backward?"=FALSE, "Right Servo"=0, "Left Servo"=0, "IR Override"=FALSE, "Intake Danger?"=FALSE}, "Intake Status Cluster"={"Roller Power"=0.0, "Angle Power"=0.0, "Intake Mode"=enum."Auto", "Intake States"=enum."Idle", "Rollers Active?"=FALSE, "Current Height"=0.0, "Target Height"=0.0, "Encoder Raw Position"=0.0, "Forward Tripped?"=FALSE, "Backward Tripped?"=FALSE, "Override IR?"=FALSE}, "Ultrasonic Data"={"Left Ultrasonic"=0.0, "Right Ultrasonic"=0.0}, "Climb Status Cluster"={"Pull Power"=0.0, "Unpin Power"=0.0, "PTO Engaged?"=FALSE, "Climb Mode"=enum."Auto"}, "Loop Times"={"DT Loop Timer"=0, "Shooter Loop Timer"=0, "Intake Loop Timer"=0, "US Loop Timer"=0, "Auton File Loop Timer"=0}, "Pressure"=0.0, "Pressure Voltage"=0.0}, binary string=w182) -> (value=w167:T54)  [unwired: 3 in, 2 out]
        n55 = Unbundle By Name(w185) -> ("Robot IP"=→"Robot IP":string, "Camera Addr"=→"Camera IP":string)
        n56 = Unbundle By Name(w167) -> ("Auton Command Cluster"=→"Auton Command Cluster":T7, "Auton File Lists"=→"Auton File Lists":T8, "Shooter State Cluster"=w158:T19, "Encoder Values"=→"Encoder Values":T14, "Drivetrain Status Cluster"=w157:T10, "IMU Data"=w151:T31, "Power and Diagnostic Data"=→"Power and Diagnostic Data":T40, "Gyro"=→"Gyro" →"Gyro 2":dbl, "Intake Status Cluster"=w166:T25, "Climb Status Cluster"=w160:T29, "Loop Times"=→"Loop Times":T48, "Ultrasonic Data"=→"Ultrasonic Data":T33, "Pressure"=→"Pressure":dbl, "Pressure Voltage"=→"Pressure Sensor Voltage":dbl)
        "IMU Data" <- w151
        "Intake Status Cluster" <- w166
        "Climb Status Cluster" <- w160
        "Shooter State Cluster" <- w158
        "Drivetrain Status Cluster" <- w157
        n57 = Unbundle By Name(w158) -> ("Right RPM"=→"Right RPM":dbl, "Left RPM"=→"Left RPM":dbl, "Angle Ready?"=→"Angle Ready?":bool, "RPM Ready?"=→"RPM Ready?":bool, "Vision Ready?"=→"Vision Ready?":bool, "Ball Loaded?"=→"Ball Loaded?":bool, "Shooter Ready?"=→"Shooter Ready?":bool, "State"=w177:T20, "Mode"=w176:T21)
        n58 = Unbundle By Name(w151) -> ("NAVX_CAL_STATUS"=→"NAVX_CAL_STATUS":T5)
        n59 = Unbundle By Name(w157) -> ("Modes"=w141:T11)
        n60 = Unbundle By Name(w166) -> ("Intake States"=w146:T27, "Intake Mode"=w163:T26)
        n61 = case shown="\"Hybrid\"" w141 {
          tunnel: ["Manual" "Climb" "Goal Target" "PID Drive" "Hybrid Drive"] -> w139
          tunnel: [u32 16711680 u32 16770560 u32 6618880 u32 9263615 u32 16743698] -> w140
          frame "Manual", Default {
          }
          frame "Climb" {
          }
          frame "Goal Vision Targeting" {
          }
          frame "PID Distance Drive" {
          }
          frame "Hybrid" {
          }
        }
        n62 = Unbundle By Name(w160) -> ("Climb Mode"=w132:T30)
        n63 = case shown="\"Shooter Ready\"" w177 {
          tunnel: ["Idle" "Warmup" "Shooter Ready" "Shooting"] -> w172
          tunnel: [u32 3381759 u32 16746240 u32 16711680 u32 6618880] -> w175
          frame "Idle", Default {
          }
          frame "Warmup" {
          }
          frame "Shooter Ready" {
          }
          frame "Shoot" {
          }
        }
        n64 = case shown="\"Move to angle\"" w146 {
          tunnel: ["Idle" "Rolling Rollers" "Moving to Angle"] -> w150
          tunnel: [u32 3381759 u32 16746240 u32 16711680] -> w149
          frame "Idle", Default {
          }
          frame "Set roller speed" {
          }
          frame "Move to angle" {
          }
        }
        n65 = case shown="\"Auto\"" w176 {
          tunnel: ["Manual" "Safe" "Auto"] -> w180
          tunnel: [u32 16711680 u32 16770560 u32 6618880] -> w181
          frame "Manual", Default {
          }
          frame "Safe" {
          }
          frame "Auto" {
          }
        }
        n66 = case shown="\"Auto\"" w132 {
          tunnel: ["Manual" "Auto"] -> w136
          tunnel: [u32 16711680 u32 6618880] -> w133
          frame "Manual", Default {
          }
          frame "Auto" {
          }
        }
        n67 = case shown="\"Safe\"" w163 {
          tunnel: ["Manual" "Safe" "Auto"] -> w161
          tunnel: [u32 16711680 u32 16770560 u32 6618880] -> w164
          frame "Manual", Default {
          }
          frame "Safe" {
          }
          frame "Auto" {
          }
        }
        n68 = Bundle(w140, w140) -> (w137:cluster{u32, u32})  [unwired: 1 in]
        n69 = Build Array(w137) -> (w138:cluster{u32, u32}[])
        n70 = Bundle(w149, w149) -> (w148:cluster{u32, u32})  [unwired: 1 in]
        n71 = Bundle(w181, w181) -> (w178:cluster{u32, u32})  [unwired: 1 in]
        n72 = Bundle(w175, w175) -> (w174:cluster{u32, u32})  [unwired: 1 in]
        n73 = Build Array(w148) -> (w147:cluster{u32, u32}[])
        n74 = Build Array(w178) -> (w179:cluster{u32, u32}[])
        n75 = Bundle(w133, w133) -> (w134:cluster{u32, u32})  [unwired: 1 in]
        n76 = Build Array(w174) -> (w173:cluster{u32, u32}[])
        n77 = property on="Drivetrain Mode" class="Bool (strict)"("BoolText.Text"=w139, "Colors [4]"=w138) -> ()  [unwired: 2 in, 2 out]
        n78 = property on="Intake State" class="Bool (strict)"("Colors [4]"=w147, "BoolText.Text"=w150) -> ()  [unwired: 2 in, 2 out]
        n79 = Bundle(w164, w164) -> (w165:cluster{u32, u32})  [unwired: 1 in]
        n80 = property on="Shooter Mode" class="Bool (strict)"("BoolText.Text"=w180, "Colors [4]"=w179) -> ()  [unwired: 2 in, 2 out]
        n81 = Build Array(w134) -> (w135:cluster{u32, u32}[])
        n82 = property on="Shooter State" class="Bool (strict)"("BoolText.Text"=w172, "Colors [4]"=w173) -> ()  [unwired: 2 in, 2 out]
        n83 = Build Array(w165) -> (w162:cluster{u32, u32}[])
        n84 = property on="Climb Mode" class="Bool (strict)"("BoolText.Text"=w136, "Colors [4]"=w135) -> ()  [unwired: 2 in, 2 out]
        n85 = property on="Intake Mode" class="Bool (strict)"("BoolText.Text"=w161, "Colors [4]"=w162) -> ()  [unwired: 2 in, 2 out]
        "Control Info" <- w188
        "Status Info" <- w187
        "Robot Metrics" <- w186
        "DS TCP" <- w185
      }
    }
  }
  n86 = while {
    stop <- FALSE stop-if-true
    n87 = local read "Goal Vision Packet"() -> (w239:T36)
    n88 = Bundle By Name(cluster=T55 {"Shooter Presets"={"Batter Shot"={"Left"=0.0, "Right"=0.0, "Angle"=0.0}, "Deep Middle Shot"={"Left"=0.0, "Right"=0.0, "Angle"=0.0}, "Manual Shot"={"Left"=0.0, "Right"=0.0, "Angle"=0.0}, "Left Ticks Per Rotation"=0.0, "Right Ticks Per Rotation"=0.0, "Low Bar Shot"={"Left"=0.0, "Right"=0.0, "Angle"=0.0}, "Shooter RPM Tolerance"=0.0, "IIR Filter Power"=0.0, "Trigger Power"=0.0, "Fire from Load Delay"=0, "Max Angle"=0.0, "Min Angle"=0.0, "Angle PID gains"={"P"=1.0, "I"=0.01, "D"=0.0}, "Angle Output"={"output high"=0.0, "output low"=0.0}, "Shooter Angle Tolerance"=0.0, "Vision Shoot x^2"=0.0, "Vision Shoot x"=0.0, "Offset Angle"=0.0, "High Goal Center Height"=97.0, "Feed Forward Max Accel"=0.0, "Feed Forward Kv"=0.0, "Backwards Trigger"=0.0, "Shot Finish Delay (ms)"=0.0, "Angle Max Current"=0.0, "Angle Current Trip Time"=0.0, "Intake Angle"=0.0, "Vision Shoot c"=0.0, "Reset?"=FALSE, "Servo Release Delay"=0.0, "Servo Idle Angle"=0, "Servo Hold Angle"=0, "Angle Pot x"=0.0, "Angle Pot c"=0.0, "Ignore Angle?"=FALSE, "Manual Output?"=FALSE, "Manual Out"=0.0, "Max RPM"=0.0, "Safty Frist Angle"=0.0, "Intake Danger Height"=0.0, "Angle Pot B"=0, "Angle Pot M"=0.0, "FF Finish RPM"=0.0, "RPM PID Right"={"P"=1.0, "I"=0.01, "D"=0.0, "FF"=0.0}, "RPM PID Left"={"P"=1.0, "I"=0.01, "D"=0.0, "FF"=0.0}, "Backwards RPM"=0.0, "Vision RPM"=0.0}, "Encoder Control"={"Right Tick Constant"=0.0, "Left Tick Constant"=0.0, "Reset?"=FALSE, "Y Dist"={"PID gains"={"proportional gain (Kc)"=0.0, "integral time (Ti, min)"=0.0, "derivative time (Td, min)"=0.0}}, "Y Stop Thresh"=0.0, "Y Stop Speed"=0.0}, "Steer PID output"={"output high"=0.0, "output low"=0.0}, " Steer PID gains"={"proportional gain (Kc)"=0.0, "integral time (Ti, min)"=0.0, "derivative time (Td, min)"=0.0}, "Drivetrain Settings"={"Gyro Tolerance"=0.0, "Throttle Ramp (ms)"=0.0, "Angular rate compensation"=FALSE, "Throttle to Rate Scale"=1.0, "Rate compensation gain"=0.01, "Kv"=0.0, "Ka"=0.0, "Feed Forward P"=0.0, "Feed Forward D"=0.0, "Goal Vision PID gains"={"proportional gain (Kc)"=1.0, "integral time (Ti, min)"=0.01, "derivative time (Td, min)"=0.0}, "Goal Detection Window"=0.0, "Creep Rate"=0.0}, "Vision Packet"={"Distance"=0.0, "Center X"=0.0, "Center Y"=0.0, "Found Target?"=FALSE, "Robot Center"=0.0, "Angle"=0.0}, "Dashboard Drivetrain Command"={"Drivetrain Vision"={"Goal Window"=0.0, "Ball Window"=0.0}}, "Info/Command Cluster"={"Distance to Ball"=0.0, "Desired Angle"=0.0, "Command"=enum."Turn to Ball", "Pixels from Center"=0.0}, "Ball Vision Packet"={"Ball Detected?"=FALSE, "Distance to Ball"=0.0, "Desired Angle"=0.0, "Pixels from Center"=0.0, "Tracking mode"=enum."Turn to Ball"}, "Intake Presets"={"Intake Speed"=0.0, "Outake Speed"=0.0, "Low Height"=0.0, "Half Height"=0.0, "Full Height"=0.0, "Angle Speed"=0.0, "Angle Tolerance"=0.0, "Encoder Scale"=0.0, "Load Height"=0.0, "Output Range"={"output high"=0.0, "output low"=0.0}, "Rotation Power Max/Min"=0.0, "MaxCurrent"=0.0, "Intake Trip Time"=0.0, "Idle Height"=0.0, "Max Height"=0.0, "Reset Encoders?"=FALSE, "PID gains"={"proportional gain (Kc)"=0.0, "integral time (Ti, min)"=0.0, "derivative time (Td, min)"=0.0}}, "Intake Encoder Control"={"Arm Tick Constant"=0.0, "Reset?"=FALSE, "Y Dist"={"PID gains"={"proportional gain (Kc)"=0.0, "integral time (Ti, min)"=0.0, "derivative time (Td, min)"=0.0}}, "Y Stop Thresh"=0.0, "Y Stop Speed"=0.0}, "Climb Presets"={"Pull Power"=0.0, "Time to Hold"=0.0, "Extend Power"=0.0}, "Goal Output Range"={"output high"=0.0, "output low"=0.0}, "Enabled Systems"={"Shoot"=TRUE, "Intake"=TRUE, "DT"=TRUE, "Gyro"=TRUE, "100ms"=TRUE, "US"=TRUE}, "Auton Presets"={"Pitch Limit"=0.0, "Roll Limit"=0.0, "Ultrasonic Limit"=0.0, "Start Position"=0.0, "Cross Position"=0.0}, "Pressure M"=0.0, "Pressure B"=0.0} ("anything"), "Shooter Presets"="Shooter Presets", "Goal Output Range"="Goal Output Range", "Vision Packet"=w239, "Drivetrain Settings"="Drivetrain Settings", "Steer PID output"="Steer PID output", "Steer PID gains"="Steer PID gains", "Intake Presets"="Intake Presets", "Climb Presets"="Climb Presets", "Encoder Control"="Encoder Settings", "Auton Presets"="Auton Presets", "Enabled Systems"="Enabled Systems", "Pressure M"="Pressure M", "Pressure B"="Pressure B") -> (w243:T55)
    n89 = Flatten To String(anything=w243) -> (data string=w245:string)  [unwired: 3 in, 2 out]
    n90 = Wait (ms)(milliseconds to wait=u32 250) -> ()  [unwired: 1 out]
    n91 = local read "Robot IP"() -> (w247:string)
    n92 = call "DumbDash Send.vi"("Robot IP"=w247, "data string"=w245) -> ()  [unwired: 10 in]
  }
  n93 = while {
    tunnel: w34 -> [w256]
    shift-right: [w248] -> _
    shift-left: w33 -> [w255]
    tunnel: [w254] -> _
    tunnel: w29 -> [w253]
    tunnel: w28 -> [w252]
    tunnel: w27 -> [_]
    tunnel: w24 -> [w251]
    shift-right: [w249] -> _
    shift-left: _ -> [w250]
    i -> [w254]
    stop <- FALSE stop-if-true
    n94 = event shown="[0] \"Rec Mode\": Value Change" {
      selector: w252 -> [_ _ _]
      dyn-events: [w260 _ _] -> _
      timeout: _ -> [_ _ _]
      tunnel: w256 -> [_ _ _]
      tunnel: w255 -> [w265 _ _]
      tunnel: w253 -> [w264 _ w278]
      tunnel: w251 -> [w263 _ _]
      tunnel: w250 -> [_ _ _]
      tunnel: [0 _ _] -> w249
      tunnel: [w265 _ _] -> w248
      event "Rec Mode": Value Change {
        n95 = event-data() -> ("NewVal"=w258:enum32{"Stop", "Record", "Playback"})  [unwired: 1 in]
        n96 = case shown="\"Playback\"" w258 {
          tunnel: w264 -> [_ w268 w272]
          tunnel: [_ _ w276] -> w260
          tunnel: [_ _ w275] -> _
          tunnel: w263 -> [_ _ w270]
          tunnel: cluster{i32, i32} {-250, 170} -> [_ _ w269]
          tunnel: [_ _ T62 {"Image Size"=TRUE, "Image Type"=TRUE, "Pixel Value"=TRUE, "ROI Information"=TRUE, "Zoom Factor"=FALSE} ("Image Information Shown:All Elements")] -> _
          tunnel: [_ _ TRUE ("Zoom Factor")] -> _
          frame Default {
          }
          frame "Stop", "Record" {
            # "Place Window too"
            n97 = invoke class="VI" method="FP.Close"(reference=w268) -> (reference out=w267:refnum<vi>)  [unwired: 2 in, 2 out]
            n98 = invoke class="VI" method="Abort VI"(reference=w267) -> ()  [unwired: 2 in, 3 out]
          }
          frame "Playback" {
            n99 = call "Open Playback Panel.vi"("Offset"=w269, "DB VI Ref"=w270, "Playback in"=w272) -> ("Playback out"=w271:refnum<vi>)  [unwired: 8 in]
            n100 = register-events(w271) -> (reference out=w276:refnum<event-registration>, error out=w275:errorcluster)  [unwired: 2 in]
          }
        }
        n101 = global write "WPI_DashboardLogging Global.vi" "Logging Filename"(path "") -> ()
        n102 = global write "WPI_DashboardLogging Global.vi" "Recording"(w258) -> ()
        n103 = call <vilib>:"WPI_DashboardNT Log FieldName Cache.vi"("Operation"=enum16{"Lookup/Add", "Index", "Clear"}."Clear") -> ()  [unwired: 8 in, 3 out]
      }
      event Panel Close {
        w277 = enum32{"Stop", "Record", "Playback"}."Stop" ("Rec Mode")
        n104 = event-data() -> ()  [unwired: 1 in, 4 out]
        n105 = local write "Rec Mode"(w277) -> ()
        n106 = global write "WPI_DashboardLogging Global.vi" "Recording"(w277) -> ()
      }
      event Panel Close {
        n107 = event-data() -> ()  [unwired: 1 in, 4 out]
        n108 = invoke class="VI" method="FP.Close"(reference=w278) -> (reference out=w280:refnum<vi>)  [unwired: 2 in, 2 out]
        n109 = invoke class="VI" method="Abort VI"(reference=w280) -> (error out=w279:errorcluster)  [unwired: 2 in, 2 out]
        n110 = invoke class="VI" method="Abort VI"(error in=w279) -> ()  [unwired: 2 in, 3 out]
      }
    }
  }
  n111 = property class="Pnl"(reference=w31) -> ("Panes[]"=w32:refnum<vi>[])  [unwired: 1 in, 2 out]
  n112 = Index Array(array=w32) -> (element=w30:refnum<vi>)  [unwired: 1 in]
  n113 = while {
    tunnel: w30 -> [w282]
    i -> [w285]
    stop <- FALSE stop-if-true
    n114 = Wait (ms)(milliseconds to wait=u32 100) -> ()  [unwired: 1 out]
    n115 = case shown="\"Record\"" "Rec Mode" {
      tunnel: w285 -> [_ _ w300]
      tunnel: [u32 2829099 ("Base Color") u32 11141120 ("Target Color") w289] -> w281
      frame "Stop", Default {
        # "Reset the color, extra updates don't cost much"
      }
      frame "Record" {
      }
      frame "Playback" {
        # "Playback"
        n116 = Quotient & Remainder(x=w300, y=u32 50 ("milliseconds to wait")) -> (x-y*floor(x/y)=w296:u32)  [unwired: 1 out]
        n117 = Divide(x=w296, y=u32 50 ("milliseconds to wait")) -> (x/y=w293:dbl)
        n118 = Multiply(x=6.283185307179586, y=w293) -> (x*y=w298:dbl)
        n119 = Sine(x=w298) -> (sin(x)=w297:dbl)
        n120 = Absolute Value(x=w297) -> (abs(x)=w290:dbl)
        n121 = call "Interpolate RGB Color.vi"("Proportion"=w290, "Target Color"=u32 30976, "Base Color"=u32 2829099) -> ("Result Color"=w289:u32)  [unwired: 8 in]
      }
    }
    n122 = property class="Pane"(reference=w282, "PaneColor"=w281) -> ()  [unwired: 1 in, 2 out]
  }
  n123 = global write "WPI_DashboardLogging Global.vi" "Recording"(w15) -> ()
  n124 = local write "Rec Mode"(w15) -> ()
  n125 = call "IMAQ Create"("Image Name"="Ball Watcher", "Image Type"=w4) -> ("New Image"=w1:T3)  [unwired: 3 in, 1 out]
  n126 = while {
    tunnel: w1 -> [w302]
    stop <- FALSE stop-if-true
    n127 = local read "Camera IP"() -> (w308:string)
    n128 = local read "Rec Mode"() -> (w309:enum32{"Stop", "Record", "Playback"})
    n129 = call "624WPI_CameraRead MJPG for Dashboard.vi"("Camera Settings"="Ball Camera Settings", "Rec Mode"=w309, "Camera IP"=w308, "Camera Mode"="Camera Mode 2", "Refnum in"=w302) -> ("Active"=w310:bool, "Refnum out"=w304:T3, "FPS"=w305:dbl, "Bandwidth (Mbps)"=w306:dbl)  [unwired: 3 in]
    "Ball Cam Active?" <- w310
    n130 = case shown="False" w310 {
      tunnel: w304 -> [_ w312]
      tunnel: w305 -> [_ w314]
      tunnel: w306 -> [_ w313]
      frame False {
        n131 = Wait Until Next ms Multiple(millisecond multiple=u32 500) -> ()  [unwired: 1 out]
      }
      frame True {
        "Front Camera Display 2" <- w312
        "FPS 2" <- w314
        "Bandwidth (Mbps) 2" <- w313
        "Front Camera Display 3" <- w312
      }
    }
  }
  n132 = while {
    tunnel: u16 1741 ("timeout ms (25000)") -> [w316]
    stop <- FALSE stop-if-true
    n133 = TCP Create Listener(10:w316) -> (0:w315:errorcluster, 3:w317:refnum<k5>)  [unwired: 4 in, 1 out]
    n134 = case shown="No Error" w315 {
      selector: w315 -> [w319 _]
      tunnel: w317 -> [w320 _]
      frame No Error {
        n135 = while {
          tunnel: w320 -> [w323]
          tunnel: w319 -> [w322]
          stop <- FALSE stop-if-true
          n136 = TCP Wait On Listener(8:w322, 11:w323) -> (0:w324:errorcluster, 4:w325:refnum<k5>)  [unwired: 2 in, 3 out]
          n137 = local write "TCP"(w325) -> ()
          n138 = case shown="No Error" w324 {
            frame No Error {
            }
            frame Error {
              n139 = Wait (ms)(milliseconds to wait=u32 1000) -> ()  [unwired: 1 out]
            }
          }
        }
      }
      frame Error {
        n140 = Wait (ms)(milliseconds to wait=u32 1000) -> ()  [unwired: 1 out]
      }
    }
  }
  n141 = call <vilib>:"Intialize Keyboard.vi"() -> ("device ID"=w14:refnum<k1>)  [unwired: 10 in, 1 out]
  n142 = while {
    stop <- FALSE stop-if-true
    n143 = local read "IMU Data"() -> (w339:T31)
    n144 = local read "Mode"() -> (w335:T4)
    n145 = Unbundle By Name(w339) -> ("Data Valid?"=w338:bool)
    n146 = Equal?(x=w335, y=T4."Disconnected") -> (x = y?=w332:bool)
    n147 = Equal?(x=w335, y=T4."No Code") -> (x = y?=w333:bool)
    n148 = Or(x=w332, y=w333) -> (x .or. y?=w334:bool)
    n149 = Or(x=w338, y=w334) -> (x .or. y?=w331:bool)
    n150 = case shown="False" w331 {
      tunnel: [w340 u32 2829099 ("Base Color")] -> w328
      frame False {
        n151 = Tick Count (ms)() -> (millisecond timer value=w341:u32)
        n152 = Quotient & Remainder(x=w341, y=u32 1000 ("milliseconds to wait")) -> (x-y*floor(x/y)=w348:u32)  [unwired: 1 out]
        n153 = Divide(x=w348, y=u32 1000 ("milliseconds to wait")) -> (x/y=w345:dbl)
        n154 = Multiply(x=6.283185307179586, y=w345) -> (x*y=w350:dbl)
        n155 = Sine(x=w350) -> (sin(x)=w349:dbl)
        n156 = Absolute Value(x=w349) -> (abs(x)=w344:dbl)
        n157 = call "Interpolate RGB Color.vi"("Proportion"=w344, "Target Color"=u32 16711680, "Base Color"=u32 2829099) -> ("Result Color"=w340:u32)  [unwired: 8 in]
      }
      frame True {
      }
    }
    n158 = property on="Gyro" class="Knob (strict)"("BGColor"=w328) -> ()  [unwired: 2 in, 2 out]
    n159 = property on="Gyro 2" class="Knob (strict)"("BGColor"=w328) -> ()  [unwired: 2 in, 2 out]
    n160 = Wait (ms)(milliseconds to wait=u32 50) -> ()  [unwired: 1 out]
  }
  n161 = while {
    tunnel: w14 -> [w357]
    stop <- FALSE stop-if-true
    n162 = local read "Robot IP"() -> (w355:string)
    n163 = call-poly <vilib>:"Acquire Input Data.vi"("device ID"=w357) -> ("keys pressed"=w356:T63)  [unwired: 16 in, 2 out]
    n164 = call "Send Keyboard Data.vi"("Robot IP"=w355, "keys pressed"=w356) -> ()  [unwired: 10 in]
    n165 = Wait (ms)(milliseconds to wait=50) -> ()  [unwired: 1 out]
  }
  n166 = global write "WPI_DashboardLogging Global.vi" "Recording"(w25) -> ()
  n167 = local write "Rec Mode"(w25) -> ()
  n168 = control-ref of="Dashboard Tab"() -> (w2:refnum<vi>)
  n169 = call "DumbDash Load Controls.vi"("TabControl in"=w2) -> ("Array"=w17:T64[])  [unwired: 10 in]
  n170 = control-ref of="DumbDashMessage"() -> (w16:refnum<vi>)
  n171 = while {
    tunnel: w17 -> [w363]
    tunnel: w16 -> [w361]
    stop <- FALSE stop-if-true
    n172 = Wait (ms)(milliseconds to wait=u32 250) -> ()  [unwired: 1 out]
    n173 = disable-structure shown="RUN_TIME_ENGINE==True" {
      disable-tunnel: "stop" -> [w366 w367]
      frame condition #0 {
        # "Close the build DB"
        n174 = Quit LabVIEW(quit? (T)=w366) -> ()
      }
      frame condition #1 (active) {
        n175 = Stop(stop? (T)=w367) -> ()
      }
    }
    n176 = case shown="True" "Save" {
      tunnel: w363 -> [_ w377]
      tunnel: w361 -> [_ w376]
      tunnel: "Robot" -> [_ w375]
      frame False {
      }
      frame True {
        n177 = flat-sequence {
          tunnel: w377 -> [w380]
          tunnel: w376 -> [w379]
          tunnel: w375 -> [w378]
          frame #0 {
            n178 = call "DumbDash Save Values.vi"("Message Box"=w379, "Robot"=w378, "Controls In"=w380) -> ()  [unwired: 9 in]
          }
          frame #1 {
            n179 = local write "Save"(FALSE) -> ()
          }
        }
      }
    }
    n180 = case shown="True" "Load" {
      tunnel: w363 -> [_ w370]
      tunnel: w361 -> [_ w369]
      tunnel: "Robot" -> [_ w368]
      frame False {
      }
      frame True {
        n181 = flat-sequence {
          tunnel: w370 -> [w373]
          tunnel: w369 -> [w372]
          tunnel: w368 -> [w371]
          frame #0 {
            n182 = call "DumbDash Load Values.vi"("Message Box"=w372, "Robot"=w371, "Controls In"=w373) -> ()  [unwired: 9 in]
          }
          frame #1 {
            n183 = local write "Load"(FALSE) -> ()
          }
        }
      }
    }
  }
  n184 = local write "Load"(TRUE) -> ()
